vi "InduceDisturbance.vi"(6 "Disturbance length\n (number of iterations)":i32, 9 "Disturbance":bool, 10 "Disturbance\nAmplitude [deg]":dbl=1.0 format="%#_13g") -> (1 "Disturbance\nAmplitude":dbl, 2 "Flag for log":dbl)   [LabVIEW 2016]
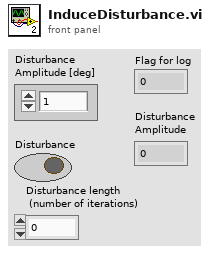
[diagram p1: front panel]
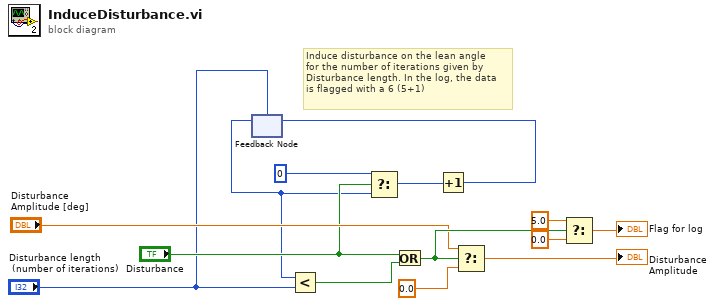
[diagram p0: block diagram]
diagram:
  # "Induce disturbance on the lean angle\nfor the number of iterations given by \nDisturbance length. In the log, the data\nis flagged with a 6 (5+1)"
  n1 = feedback #1("Disturbance length\n (number of iterations)") -> (w2:i32)
  n2 = Less?(x=w2, y="Disturbance length\n (number of iterations)") -> (x < y?=w5:bool)
  n3 = Select(t=0, s="Disturbance", f=w2) -> (s? t:f=w10:i32)
  n4 = Or(x="Disturbance", y=w5) -> (x .or. y?=w11:bool)
  n5 = Increment(x=w10) -> (x+1=w3:i32)
  n6 = feedback-in #1(w3) -> ()
  n7 = Select(t="Disturbance\nAmplitude [deg]", s=w11, f=0.0 ("Disturbance\nAmplitude")) -> (s? t:f=→"Disturbance\nAmplitude":dbl)
  n8 = Select(t=5.0, s=w11, f=0.0) -> (s? t:f=→"Flag for log":dbl)
